vi "Build_Write File Record.vi"(0 "File Number":u16, 1 "Record Number":u16, 2 "values":u16[](array[numeric]), 3 "error in (no error)":errorcluster) -> (7 "MB_PDU":T1={"Function Code"=1, "Data"=[], "RTU_DataBytes"=0}, 10 "error out":errorcluster)   [LabVIEW 2016, in "斯坦道总氮.lvlib"]
uses:
  <vilib>/Plasmionique/MB Master/MB_PDU/MB_PDU_Cluster.ctl
  <vilib>/Plasmionique/MB Master/MB Master.lvlib
panel:
  out "添加的数组":u16[](array[numeric]) format="%x"
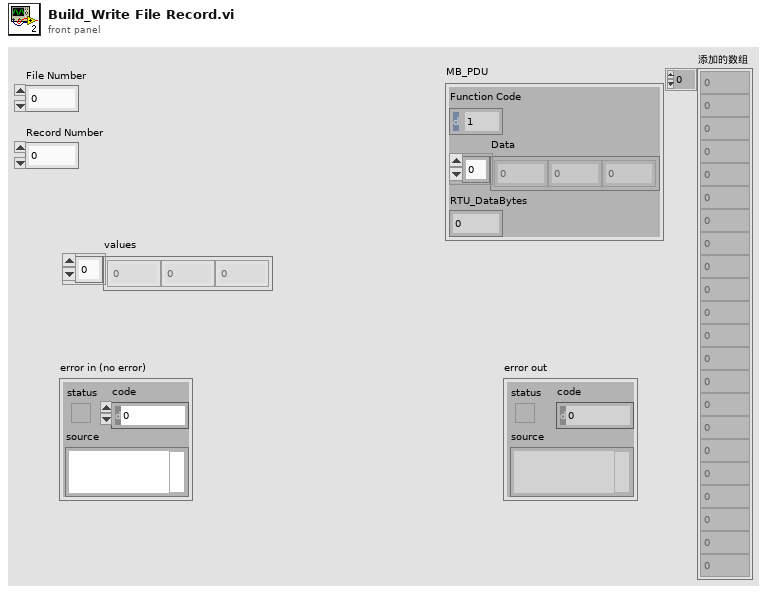
[diagram p1: front panel]
types:
  T1 = typedef "MB Master.lvlib/MB_PDU_Cluster.ctl" = cluster{"Function Code":u8, "Data":u8[], "RTU_DataBytes":i32}
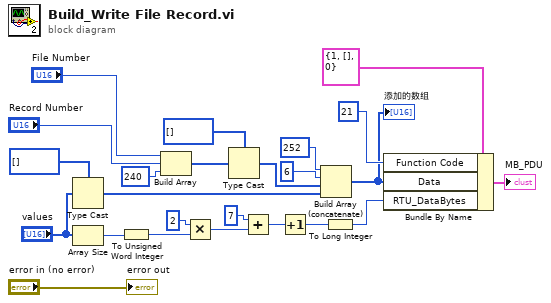
[diagram p0: block diagram]
diagram:
  n1 = Type Cast(type=u8[] [], x="values") -> (*(type *) &x=w16:u8[])
  n2 = Array Size(array="values") -> (size(s)=w13:i32)
  n3 = To Unsigned Word Integer(number=w13) -> (unsigned 16bit integer=w4:u16)
  n4 = Build Array("File Number", "Record Number", u16 240 ("元素")) -> (w24:u16[])
  n5 = Multiply(x=u16 2, y=w4) -> (x*y=w3:u16)
  n6 = Type Cast(type=u8[] [], x=w24) -> (*(type *) &x=w18:u8[])
  n7 = Add(x=u8 7, y=w3) -> (x+y=w8:u16)
  n8 = Increment(x=w8) -> (x+1=w7:u16)
  n9 = Build Array (concatenate)(u16 252 ("元素"), u8 6 ("元素"), w18, w16) -> (w15:u16[])
  "添加的数组" <- w15
  n10 = To Long Integer(number=w7) -> (32bit integer=w6:i32)
  n11 = Bundle By Name(cluster=T1 {"Function Code"=1, "Data"=[], "RTU_DataBytes"=0} ("Modbus Serial New.lvlib:MB_PDU.lvclass"), "Function Code"=u8 21, "Data"=w15, "RTU_DataBytes"=w6) -> (→"MB_PDU":T1)
  "error out" <- "error in (no error)"
